vi "Spawn.vi"(6 "Transport":refnum<class "Transport.lvclass">, 9 "UID":string, 10 "Actor":refnum<class "Actor.lvclass">, 11 "Actor in":refnum<class "Actor.lvclass">) -> (0 "Error out":errorcluster, 3 "Actor out":refnum<class "Actor.lvclass">)   [LabVIEW 2025, in "jettl.lvlib" / "Actor.lvlib" / "Actor.lvclass"]
uses:
  Actor.lvclass
  Transport/Transport/Transport.lvclass
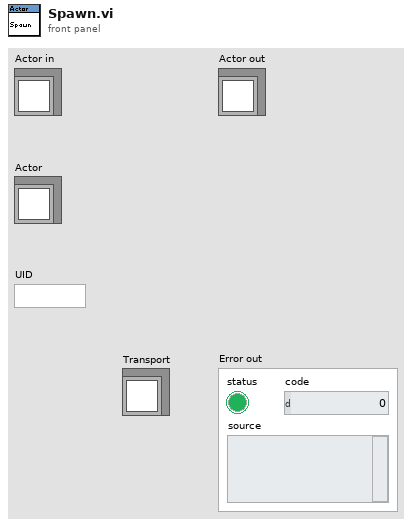
[diagram p1: front panel]
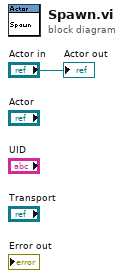
[diagram p0: block diagram]
diagram:
  "Actor out" <- "Actor in"
